vi "Read fs_px.vi"(8 "error in (no error)":errorcluster, 11 "Analyze Parameter Temporal Calibration in":refnum<class "Analyze Parameter Temporal Calibration.lvclass">) -> (0 "error out":errorcluster, 2 "fs/px":dbl[unit], 3 "Analyze Parameter Temporal Calibration out":refnum<class "Analyze Parameter Temporal Calibration.lvclass">)   [LabVIEW 2014, in "Analyze Parameter Temporal Calibration.lvclass"]
uses:
  Analyze Parameter Temporal Calibration.lvclass
  Analyze Parameter Temporal Calibration.lvclass/Analyze Parameter Temporal Calibration.ctl
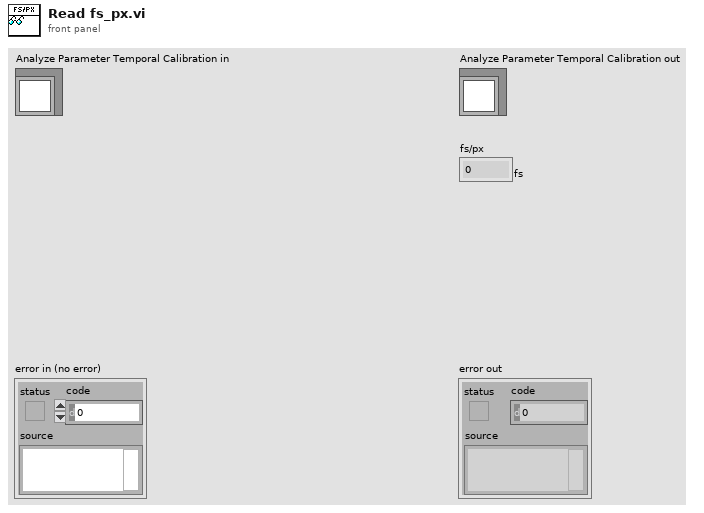
[diagram p1: front panel]
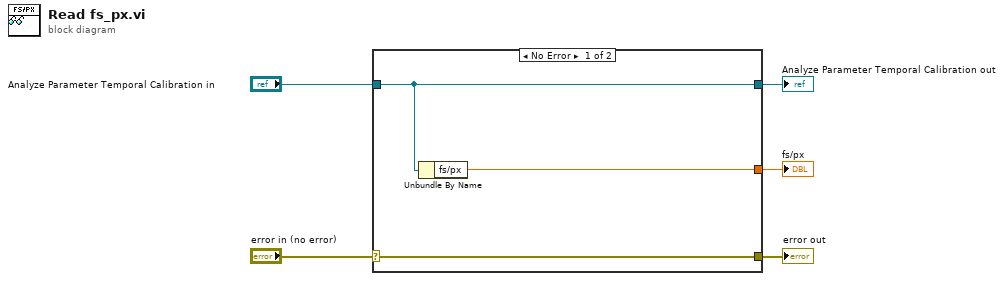
[diagram p0: block diagram]
diagram:
  n1 = case shown="No Error" "error in (no error)" {
    selector: "error in (no error)" -> [w8 w9]
    tunnel: [w8 w9] -> w4
    tunnel: [w7 w10] -> w2
    tunnel: "Analyze Parameter Temporal Calibration in" -> [w7 w10]
    tunnel: [w6 _] -> w1
    frame No Error {
      n2 = Unbundle By Name(w7) -> ("fs/px"=w6:dbl[unit])
    }
    frame Error {
    }
  }
  "error out" <- w4
  "Analyze Parameter Temporal Calibration out" <- w2
  "fs/px" <- w1
